vi "Data_conv_VI.vi"(0 "data[2]":u8, 1 "Numeric 10":dbl, 2 "data[3]":u8, 3 "data[4]":u8, 4 "data[5]":u8, 5 "data[6]":u8, 6 "data[7]":u8, 8 "Sel_1":bool, 9 "Count per volt":dbl, 10 "Sel_2":bool, 11 "Numeric 12":dbl, 12 "Numeric 6":dbl, 13 "Numeric 11":dbl, 14 "Numeric 7":dbl, 16 "Numeric 9":dbl) -> (18 "Numeric 8":dbl, 20 "Numeric 2":dbl, 21 "Numeric":dbl, 22 "Numeric 3":dbl, 23 "Numeric 4":dbl, 24 "Numeric 5":dbl)   [LabVIEW 2016]
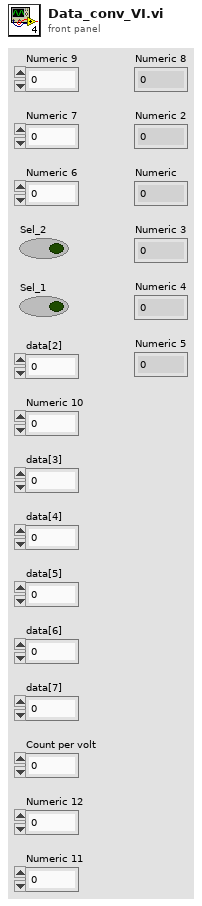
[diagram p1: front panel]
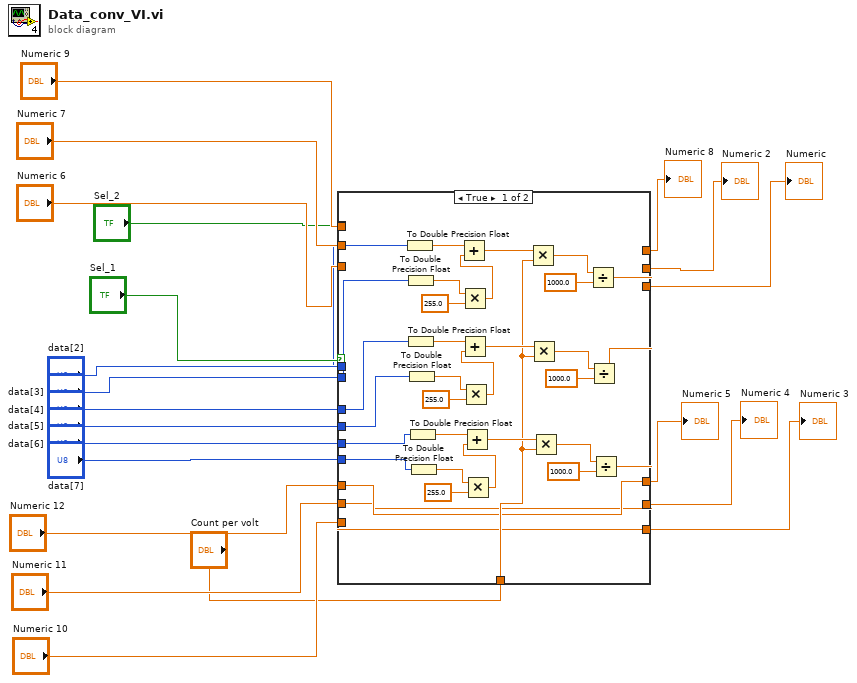
[diagram p0: block diagram]
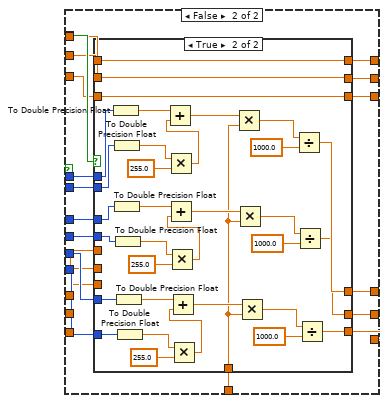
[diagram p2: hidden frame]
diagram:
  n1 = case shown="True" "Sel_1" {
    tunnel: "Sel_2" -> [_ w75]
    tunnel: "Count per volt" -> [w29 w74]
    tunnel: "data[2]" -> [w35 w73]
    tunnel: "data[3]" -> [w34 w72]
    tunnel: "data[4]" -> [w33 w71]
    tunnel: "data[5]" -> [w32 w70]
    tunnel: "data[6]" -> [w31 w69]
    tunnel: "data[7]" -> [w30 w68]
    tunnel: [w25 w67] -> w17
    tunnel: [w24 w66] -> w18
    tunnel: [w23 w65] -> w19
    tunnel: "Numeric 12" -> [w25 w64]
    tunnel: "Numeric 11" -> [w24 w63]
    tunnel: "Numeric 10" -> [w23 w62]
    tunnel: "Numeric 9" -> [_ w61]
    tunnel: [w28 w60] -> w13
    tunnel: [w27 w59] -> w20
    tunnel: "Numeric 7" -> [_ w58]
    tunnel: "Numeric 6" -> [_ w57]
    tunnel: [w26 w56] -> w21
    frame True {
      n2 = To Double Precision Float(number=w35) -> (double precision float=w41:dbl)
      n3 = To Double Precision Float(number=w34) -> (double precision float=w42:dbl)
      n4 = To Double Precision Float(number=w33) -> (double precision float=w48:dbl)
      n5 = To Double Precision Float(number=w32) -> (double precision float=w49:dbl)
      n6 = To Double Precision Float(number=w31) -> (double precision float=w54:dbl)
      n7 = To Double Precision Float(number=w30) -> (double precision float=w55:dbl)
      n8 = Multiply(x=w42, y=255.0) -> (x*y=w39:dbl)
      n9 = Add(x=w41, y=w39) -> (x+y=w37:dbl)
      n10 = Multiply(x=w49, y=255.0) -> (x*y=w46:dbl)
      n11 = Add(x=w48, y=w46) -> (x+y=w44:dbl)
      n12 = Multiply(x=w55, y=255.0) -> (x*y=w53:dbl)
      n13 = Add(x=w54, y=w53) -> (x+y=w51:dbl)
      n14 = Multiply(x=w37, y=w29) -> (x*y=w38:dbl)
      n15 = Multiply(x=w44, y=w29) -> (x*y=w45:dbl)
      n16 = Multiply(x=w51, y=w29) -> (x*y=w52:dbl)
      n17 = Divide(x=w38, y=1000.0) -> (x/y=w28:dbl)
      n18 = Divide(x=w45, y=1000.0) -> (x/y=w27:dbl)
      n19 = Divide(x=w52, y=1000.0) -> (x/y=w26:dbl)
    }
    frame False {
      n20 = case shown="True" w75 {
        tunnel: w74 -> [_ w82]
        tunnel: w73 -> [_ w110]
        tunnel: w72 -> [_ w107]
        tunnel: w71 -> [_ w92]
        tunnel: w70 -> [_ w91]
        tunnel: w69 -> [_ w90]
        tunnel: w68 -> [_ w89]
        tunnel: [w78 w88] -> w67
        tunnel: [w77 w87] -> w66
        tunnel: [w76 w86] -> w65
        tunnel: w64 -> [w78 _]
        tunnel: w63 -> [w77 _]
        tunnel: w62 -> [w76 _]
        tunnel: w61 -> [w81 w85]
        tunnel: [w81 w85] -> w60
        tunnel: [w80 w84] -> w59
        tunnel: w58 -> [w80 w84]
        tunnel: [w79 w83] -> w56
        tunnel: w57 -> [w79 w83]
        frame False {
        }
        frame True {
          n21 = To Double Precision Float(number=w110) -> (double precision float=w109:dbl)
          n22 = To Double Precision Float(number=w107) -> (double precision float=w108:dbl)
          n23 = To Double Precision Float(number=w92) -> (double precision float=w101:dbl)
          n24 = To Double Precision Float(number=w91) -> (double precision float=w100:dbl)
          n25 = To Double Precision Float(number=w90) -> (double precision float=w94:dbl)
          n26 = To Double Precision Float(number=w89) -> (double precision float=w93:dbl)
          n27 = Multiply(x=w108, y=255.0) -> (x*y=w112:dbl)
          n28 = Add(x=w109, y=w112) -> (x+y=w114:dbl)
          n29 = Multiply(x=w100, y=255.0) -> (x*y=w103:dbl)
          n30 = Add(x=w101, y=w103) -> (x+y=w105:dbl)
          n31 = Multiply(x=w93, y=255.0) -> (x*y=w96:dbl)
          n32 = Add(x=w94, y=w96) -> (x+y=w98:dbl)
          n33 = Multiply(x=w114, y=w82) -> (x*y=w113:dbl)
          n34 = Multiply(x=w105, y=w82) -> (x*y=w104:dbl)
          n35 = Multiply(x=w98, y=w82) -> (x*y=w97:dbl)
          n36 = Divide(x=w113, y=1000.0) -> (x/y=w88:dbl)
          n37 = Divide(x=w104, y=1000.0) -> (x/y=w87:dbl)
          n38 = Divide(x=w97, y=1000.0) -> (x/y=w86:dbl)
        }
      }
    }
  }
  "Numeric" <- w21
  "Numeric 2" <- w20
  "Numeric 3" <- w19
  "Numeric 4" <- w18
  "Numeric 5" <- w17
  "Numeric 8" <- w13
